vi "Kinesis generic motor benchtop stepper.vi"() -> ()   [LabVIEW 2011]
uses:
  C:/Users/nbayconich/Documents/Kinesis labview project Nick test/Thorlabs.MotionControl.Controls.dll
  Thorlabs.MotionControl.Controls.dll
  C:/Users/nbayconich/Documents/Kinesis labview project Nick test/Thorlabs.MotionControl.Benchtop.StepperMotorCLI.dll
  Thorlabs.MotionControl.Benchtop.StepperMotorCLI.dll
  C:/Users/nbayconich/Documents/Kinesis labview project Nick test/Thorlabs.MotionControl.GenericMotorCLI.dll
  Thorlabs.MotionControl.GenericMotorCLI.dll
panel:
  in  "position":dbl
  in  "Boolean":bool
  in  "stop":bool
  in  "BenchtopStepperControl":refnum<k24>(container)
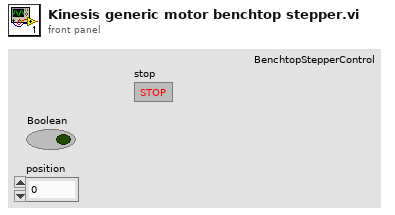
[diagram p1: front panel]
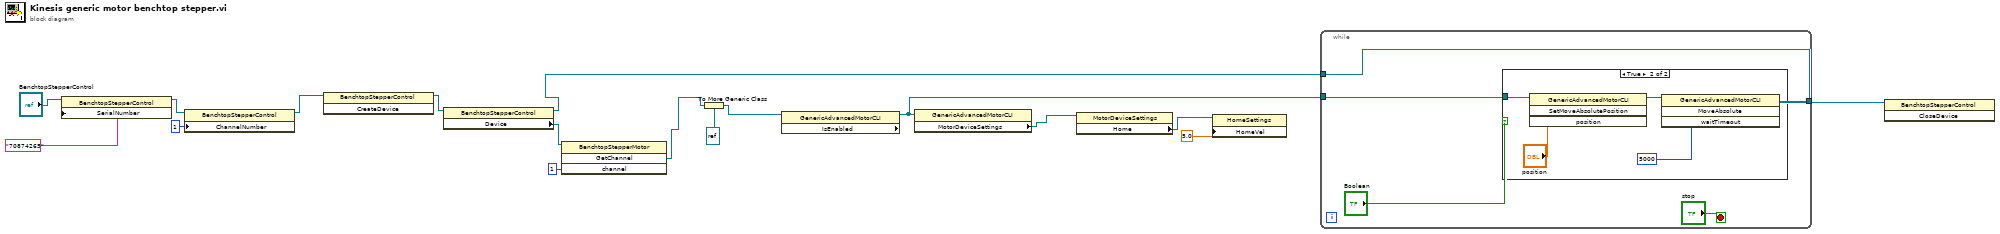
[diagram p0: block diagram]
diagram:
  n1 = property class="BenchtopStepperControl"(reference="BenchtopStepperControl", "SerialNumber"="70874265") -> (reference out=w16:refnum<k24>)  [unwired: 1 in, 1 out]
  n2 = property class="BenchtopStepperControl"(reference=w16, "ChannelNumber"=1) -> (reference out=w15:refnum<k24>)  [unwired: 1 in, 1 out]
  n3 = invoke class="BenchtopStepperControl" method="CreateDevice"(reference=w15) -> (reference out=w12:refnum<k24>)  [unwired: 2 in, 2 out]
  n4 = property class="BenchtopStepperControl"(reference=w12) -> (reference out=w10:refnum<k24>, "Device"=w11:refnum<k24>)  [unwired: 1 in, 1 out]
  n5 = invoke class="BenchtopStepperMotor" method="GetChannel"(reference=w11, "channel"=i16 1) -> ("GetChannel"=w8:refnum<k24>)  [unwired: 2 in, 3 out]
  n6 = To More Generic Class(target class=refnum<k24> refnum, reference=w8) -> (generic class reference=w7:refnum<k24>)
  n7 = property class="GenericAdvancedMotorCLI" props=["IsEnabled"](reference=w7) -> (reference out=w2:refnum<k24>)  [unwired: 1 in, 2 out]
  n8 = property class="GenericAdvancedMotorCLI"(reference=w2) -> ("MotorDeviceSettings"=w4:refnum<k24>)  [unwired: 1 in, 2 out]
  n9 = property class="MotorDeviceSettings"(reference=w4) -> ("Home"=w3:refnum<k24>)  [unwired: 1 in, 2 out]
  n10 = property class="HomeSettings"(reference=w3, "HomeVel"=5.0 ("HomeZeroOffset")) -> ()  [unwired: 1 in, 2 out]
  n11 = while {
    tunnel: [w20] -> w13
    tunnel: w10 -> [w20]
    tunnel: w2 -> [w18]
    stop <- "stop" stop-if-true
    n12 = case shown="True" "Boolean" {
      tunnel: w18 -> [_ w23]
      frame False {
      }
      frame True {
        n13 = invoke class="GenericAdvancedMotorCLI" method="SetMoveAbsolutePosition"(reference=w23, "position"="position") -> (reference out=w25:refnum<k24>)  [unwired: 2 in, 3 out]
        n14 = invoke class="GenericAdvancedMotorCLI" method="MoveAbsolute"(reference=w25, "waitTimeout"=5000) -> ()  [unwired: 2 in, 4 out]
      }
    }
  }
  n15 = invoke class="BenchtopStepperControl" method="CloseDevice"(reference=w13) -> ()  [unwired: 2 in, 3 out]
